vi "Log_Append.vi"(2 "Char Size":i32, 5 "To Front(t) End(f)":bool, 7 "Seperator":string="\r\n", 10 "Sting To Append":string, 11 "String":string) -> (3 "String Out":string)   [LabVIEW 2020]
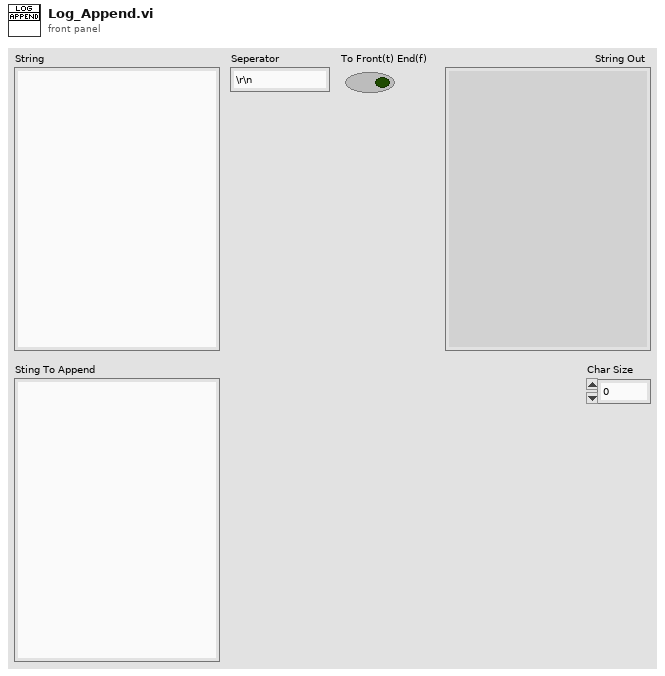
[diagram p1: front panel]
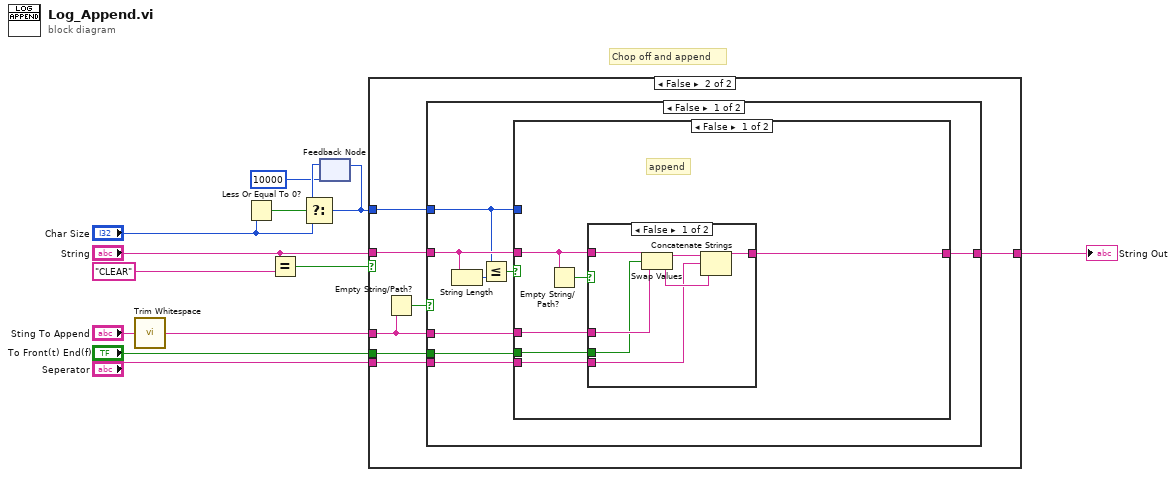
[diagram p0: block diagram]
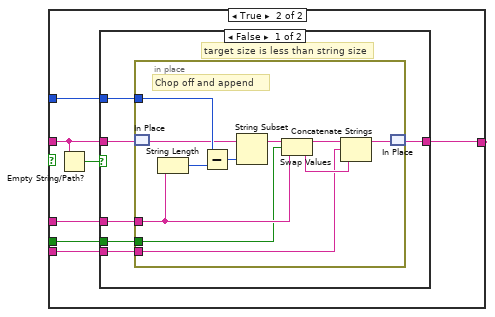
[diagram p4: hidden frame]
diagram:
  # "Chop off and append"
  n1 = call <vilib>:"Trim Whitespace.vi"("string"="Sting To Append") -> ("trimmed string"=w3:string)  [unwired: 1 in]
  n2 = Less Or Equal To 0?(x="Char Size") -> (x <= 0?=w11:bool)
  n3 = Equal?(x="String", y="CLEAR") -> (x = y?=w1:bool)
  n4 = feedback #1(10000 ("Char Size")) -> (w8:i32)
  n5 = Select(t=w8, s=w11, f="Char Size") -> (s? t:f=w9:i32)
  n6 = feedback-in #1(w9) -> ()
  n7 = case shown="False" w1 {
    tunnel: "String" -> [_ w20]
    tunnel: [_ w19] -> w12
    tunnel: w3 -> [_ w16]
    tunnel: w9 -> [_ w18]
    tunnel: "To Front(t) End(f)" -> [_ w17]
    tunnel: "Seperator" -> [_ w14]
    frame True {
      # "CLEAR"
    }
    frame False {
      n8 = Empty String/Path?(string/path=w16) -> (empty?=w15:bool)
      n9 = case shown="False" w15 {
        tunnel: w20 -> [w28 w68]
        tunnel: [w27 w68] -> w19
        tunnel: w18 -> [w25 _]
        tunnel: w17 -> [w23 _]
        tunnel: w16 -> [w22 _]
        tunnel: w14 -> [w21 _]
        frame False {
          n10 = String Length(string=w28) -> (length=w26:i32)
          n11 = Less Or Equal?(x=w25, y=w26) -> (x <= y?=w24:bool)
          n12 = case shown="False" w24 {
            tunnel: w28 -> [w31 w45]
            tunnel: w22 -> [w34 w49]
            tunnel: [w33 w48] -> w27
            tunnel: w25 -> [_ w47]
            tunnel: w23 -> [w32 w46]
            tunnel: w21 -> [w29 w43]
            frame False {
              # "append"
              n13 = Empty String/Path?(string/path=w31) -> (empty?=w30:bool)
              n14 = case shown="False" w30 {
                tunnel: w34 -> [w39 w42]
                tunnel: [w38 w42] -> w33
                tunnel: w32 -> [w37 _]
                tunnel: w31 -> [w36 _]
                tunnel: w29 -> [w35 _]
                frame False {
                  n15 = Swap Values(12:w36, 13:w37, 14:w39) -> (1:w41:string, 3:w40:string)
                  n16 = Concatenate Strings(w41, w35, w40) -> (w38:string)
                }
                frame True {
                }
              }
            }
            frame True {
              n17 = Empty String/Path?(string/path=w45) -> (empty?=w44:bool)
              n18 = case shown="False" w44 {
                tunnel: w49 -> [w55 w67]
                tunnel: w45 -> [w54 _]
                tunnel: [w53 w67] -> w48
                tunnel: w47 -> [w52 _]
                tunnel: w46 -> [w51 _]
                tunnel: w43 -> [w50 _]
                frame False {
                  # "target size is less than string size"
                  n19 = in-place {
                    in-place-border: w55 -> [w59]
                    in-place-border: w52 -> [w66]
                    in-place-border: w51 -> [w57]
                    in-place-border: w50 -> [w56]
                    # "Chop off and append"
                    n20 = in-place-match #2(w54) -> (w63:string)
                    n21 = String Length(string=w59) -> (length=w65:i32)
                    n22 = Subtract(x=w66, y=w65) -> (x-y=w64:i32)
                    n23 = String Subset(string=w63, length (rest)=w64) -> (substring=w61:string)  [unwired: 1 in]
                    n24 = Swap Values(12:w61, 13:w57, 14:w59) -> (1:w60:string, 3:w58:string)
                    n25 = Concatenate Strings(w60, w56, w58) -> (w62:string)
                    n26 = in-place-match #2(w62) -> (w53:string)
                  }
                }
                frame True {
                }
              }
            }
          }
        }
        frame True {
        }
      }
    }
  }
  "String Out" <- w12
